vi "Send Message.vi"(6 "Message Priority":enum16{"Normal", "High"}(ring), 8 "error in":errorcluster, 10 "Message Payload in":refnum<class "IMessagePayload.lvclass">, 11 "UserEventMessageTransport":refnum<class "UserEventMessageTransport.lvclass">) -> (0 "error out":errorcluster, 3 "UserEventMessageTransport":refnum<class "UserEventMessageTransport.lvclass">)   [LabVIEW 2016, in "UserEventMessageTransport.lvclass"]
uses:
  UserEventMessageTransport.lvclass
  IMessagePayload/IMessagePayload.lvclass
  <vilib>/event_ctls.llb/usereventprio.ctl
panel:
  # "INPUTS"
  # "OUTPUTS"
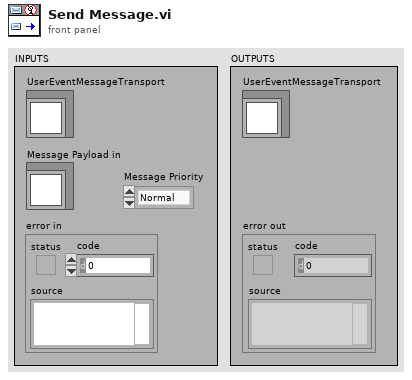
[diagram p1: front panel]
types:
  T1 = typedef "usereventprio.ctl" = enum32{"high priority", "normal priority"}
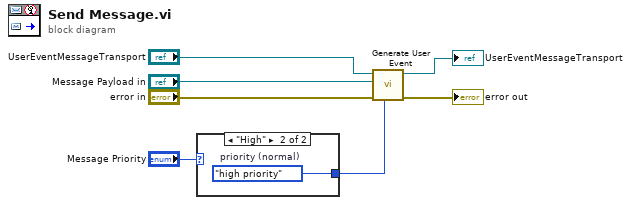
[diagram p0: block diagram]
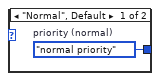
[diagram p2: hidden frame]
diagram:
  n1 = case shown="\"High\"" "Message Priority" {
    tunnel: [w8 w9] -> w3
    frame "Normal", Default {
      w8 = usereventprio."normal priority"  # priority (normal)
    }
    frame "High" {
      w9 = usereventprio."high priority"  # priority (normal)
    }
  }
  n2 = call "Generate User Event.vi"("priority (normal)"=w3, "error in"="error in", "IMessagePayload.lvclass"="Message Payload in", "UserEventMessageTransport"="UserEventMessageTransport") -> ("error out"=→"error out":errorcluster, "UserEventMessageTransport"=→"UserEventMessageTransport":refnum<class "UserEventMessageTransport.lvclass">)  [unwired: 6 in]
